vi "Set Probe Param Arrays.vi"(10 "Probe Param Array":T1[](array[typedef]) {"Sensor Block"."SensorCfgParams Array"."CalibrCoefArray" format="%#.12g"}) -> ()   [LabVIEW 2015, in "Tool Cfg.lvlib"]
uses:
  Tool Cfg.lvlib
  _ProbeConfigParams Cluster--typedef.ctl
  _Sensor Block Cluster--typedef.ctl
  _SensorConfigParams Cluster--typedef.ctl
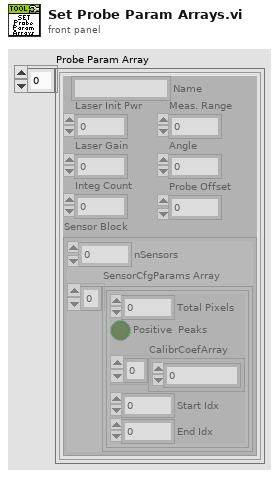
[diagram p1: front panel]
types:
  T1 = typedef "Tool Cfg.lvlib/_ProbeConfigParams Cluster--typedef.ctl" = cluster{"Name":string, "Laser Init Pwr":u16, "Laser Gain":u8, "Integ Count":u16, "Meas. Range":sgl, "Angle":sgl, "Probe Offset":sgl, "Sensor Block":T2}
  T2 = typedef "Tool Cfg.lvlib/_Sensor Block Cluster--typedef.ctl" = cluster{"nSensors":u16, "SensorCfgParams Array":T3[]}
  T3 = typedef "Tool Cfg.lvlib/_SensorConfigParams Cluster--typedef.ctl" = cluster{"Total Pixels":u16, "Positive  Peaks":bool, "CalibrCoefArray":dbl[], "Start Idx":u16, "End Idx":u16}
  T4 = typedef "Tool Cfg.lvlib/_Probe Block Cluster--typedef.ctl" = cluster{"nProbes":u16, "Probe Param Array":T1[]}
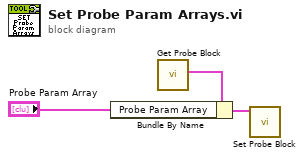
[diagram p0: block diagram]
diagram:
  n1 = call "Get Probe Block.vi"() -> ("Probe Block"=w3:T4)  [unwired: 11 in]
  n2 = Bundle By Name(cluster=w3, "Probe Param Array"="Probe Param Array") -> (w2:T4)
  n3 = call "Set Probe Block.vi"("Probe Block"=w2) -> ()  [unwired: 11 in]
